vi "WPI_AnalogChannelGetLSBWeight.vi"(8 "error in (no error)":errorcluster, 11 "AIDeviceRef":T1={"DevStatus"={"status"=FALSE, "code"=0, "source"=""}, "Analog Channel"=enum."AI 1"}) -> (0 "error out":errorcluster, 2 "LSBWeight":dbl, 3 "AIDeviceRef":T1={"DevStatus"={"status"=FALSE, "code"=0, "source"=""}, "Analog Channel"=enum."AI 1"})   [LabVIEW 2017]
doc: "Returns the least significant bit (LSB) weight constant that the A/D converter uses to scale the signal.\n\nThis software is licensed. Open the labview\\readme\\WPI Robotics Library Open Source License.txt file for more information."
uses:
  <vilib>/Rock Robotics/WPI/AnalogChannel/WPI_AnalogChannelDevRef.ctl
  <vilib>/Rock Robotics/SystemInterfaces/AI/FPGA_AIChannel.ctl
  <vilib>/Rock Robotics/SystemInterfaces/System/FPGA_SystemGet.vi
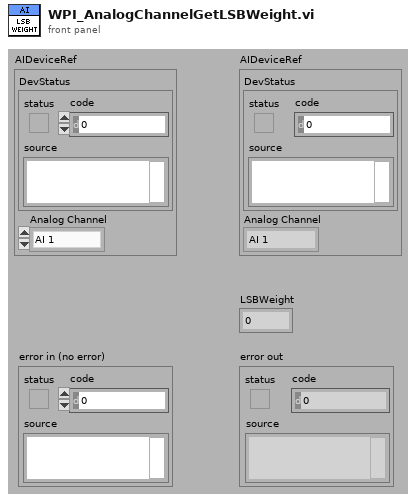
[diagram p1: front panel]
types:
  T1 = typedef "WPI_AnalogChannelDevRef.ctl" = cluster{"DevStatus":errorcluster, "Analog Channel":T2}
  T2 = typedef "FPGA_AIChannel.ctl" = enum8{"AI 0", "AI 1", "AI 2", "AI 3", "AI MXP 0", "AI MXP 1", "AI MXP 2", "AI MXP 3", "Invalid"}
  T3 = typedef "FPGA_AIDevRef.ctl" = cluster{"DevStatus":errorcluster}
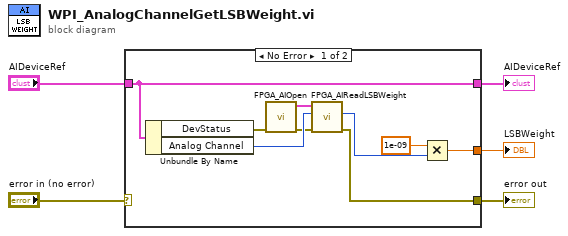
[diagram p0: block diagram]
diagram:
  n1 = case shown="No Error" "error in (no error)" {
    selector: "error in (no error)" -> [_ w15]
    tunnel: "AIDeviceRef" -> [w13 w16]
    tunnel: [w13 w16] -> w4
    tunnel: [w8 _] -> w3
    tunnel: [w9 w15] -> w1
    frame No Error {
      n2 = Unbundle By Name(w13) -> ("DevStatus"=w14:errorcluster, "Analog Channel"=w10:T2)
      n3 = call <vilib>:"FPGA_AIOpen.vi"("error in (no error)"=w14) -> ("error out"=w6:errorcluster, "AI Reference out"=w12:T3)  [unwired: 2 in, 7 out]
      n4 = call <vilib>:"FPGA_AIReadLSBWeight.vi"("error in (no error)"=w6, "Channel"=w10, "AI Reference"=w12) -> ("error out"=w9:errorcluster, "LSBWeight"=w11:u32)  [unwired: 7 out]
      n5 = Multiply(x=1e-09, y=w11) -> (x*y=w8:dbl)
    }
    frame Error {
    }
  }
  "AIDeviceRef" <- w4
  "LSBWeight" <- w3
  "error out" <- w1
